vi "CAN_init.vi"(6 "error in":errorcluster, 8 "Maximum Output Voltage":dbl=5.0, 9 "Control Mode":T3=enum."Position") -> (0 "error out":errorcluster, 3 "CAN Jaguars Ref":T1)   [LabVIEW 2009, in "OWNCAN.lvlib"]
doc: "Initializes CAN interface for both Jaguars. Sets the default settings for controller parameters and enables corresponding control mode.\nThis VI must be called at the beginning of the program before using of any CAN functionality."
uses:
  OWNCAN.lvlib
  CAN/SubVIs/CAN Jaguar Control Mode.ctl
  CAN Jaguars Ref.ctl
  CAN/SubVIs/CAN Jaguar Ref.ctl
  CAN/SubVIs/CAN Jaguar Position Reference.ctl
  Serial.lvlib
  CAN.lvlib
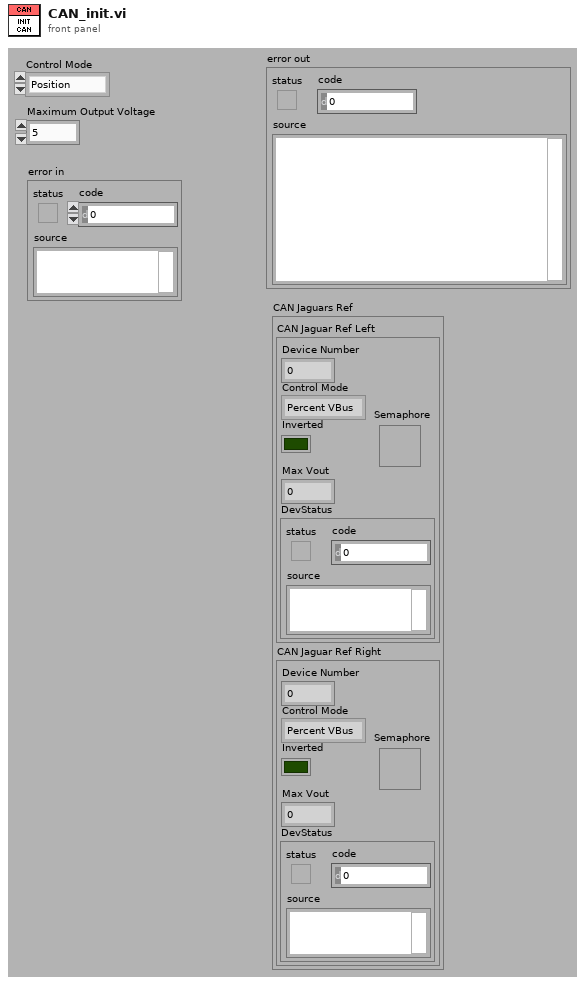
[diagram p1: front panel]
types:
  T1 = typedef "OWNCAN.lvlib/CAN Jaguars Ref.ctl" = cluster{"CAN Jaguar Ref Left":T2, "CAN Jaguar Ref Right":T2}
  T2 = typedef "CAN.lvlib/CAN Jaguar Ref.ctl" = cluster{"Device Number":u8, "Control Mode":T3, "Inverted":bool, "Semaphore":T4, "Max Vout":dbl, "DevStatus":errorcluster}
  T3 = typedef "CAN.lvlib/CAN Jaguar Control Mode.ctl" = enum16{"Percent VBus", "Speed", "Position", "Current"}
  T4 = typedef "Semaphore RefNum" = refnum<k1>
  T5 = typedef "CAN.lvlib/CAN Jaguar Position Reference.ctl" = enum16{"Encoder", "Potentiometer"}
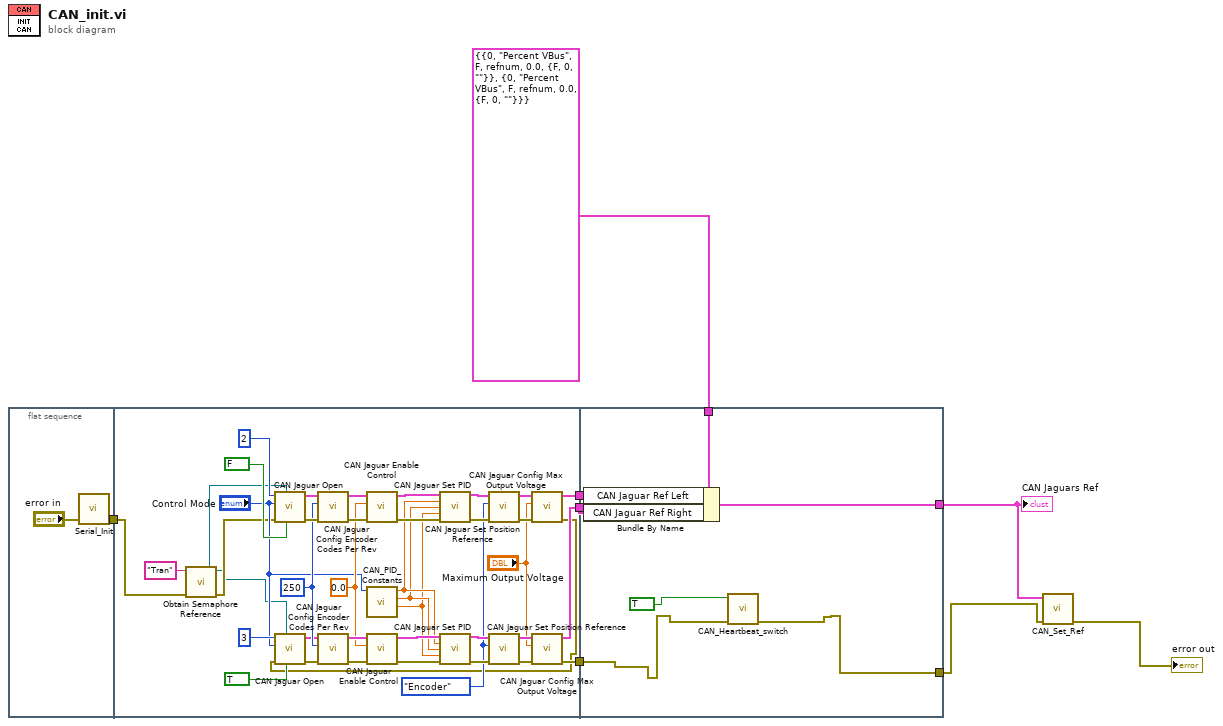
[diagram p0: block diagram]
diagram:
  n1 = flat-sequence {
    tunnel: [w9] -> w8
    tunnel: w8 -> [w15]
    tunnel: [w26] -> w7
    tunnel: [w25] -> w6
    tunnel: [w24] -> w5
    tunnel: w7 -> [w52]
    tunnel: w6 -> [w56]
    tunnel: w5 -> [w57]
    tunnel: [w55] -> w3
    tunnel: T1 {"CAN Jaguar Ref Left"={"Device Number"=0, "Control Mode"=enum."Percent VBus", "Inverted"=FALSE, "Semaphore"=refnum, "Max Vout"=0.0, "DevStatus"={"status"=FALSE, "code"=0, "source"=""}}, "CAN Jaguar Ref Right"={"Device Number"=0, "Control Mode"=enum."Percent VBus", "Inverted"=FALSE, "Semaphore"=refnum, "Max Vout"=0.0, "DevStatus"={"status"=FALSE, "code"=0, "source"=""}}} ("CAN Jaguars Ref") -> [w54]
    tunnel: [w51] -> w2
    frame #0 {
      n2 = call "Serial_Init.vi"("error in (no error)"="error in") -> ("error out"=w9:errorcluster)  [unwired: 3 in, 1 out]
    }
    frame #1 {
      w32 = 0.0 ("Encoder Initial Position")
      w33 = CAN_Jaguar_Position_Reference."Encoder" ("Position Reference")
      w46 = u16 250 ("Encoder Codes Per Rev")
      n3 = call <vilib>:"Obtain Semaphore Reference.vi"("error in (no error)"=w15, "name (unnamed)"="Tran") -> ("error out"=w14:errorcluster, "semaphore"=w11:T4)  [unwired: 3 in, 1 out]
      n4 = call "CAN Jaguar Open.vi"("Inverted"=FALSE, "Semaphore"=w11, "error in (no error)"=w14, "Control Mode"="Control Mode", "Device Number"=u8 2) -> ("error out"=w47:errorcluster, "CAN Jaguar Ref Out"=w12:T2)  [unwired: 5 in]
      n5 = call "CAN Jaguar Config Encoder Codes Per Rev.vi"("error in (no error)"=w47, "Encoder Codes Per Rev"=w46, "CAN Jaguar Ref"=w12) -> ("error out"=w43:errorcluster, "CAN Jaguar Ref Out"=w42:T2)  [unwired: 7 in]
      n6 = call "CAN Jaguar Enable Control.vi"("error in (no error)"=w43, "Encoder Initial Position"=w32, "CAN Jaguar Ref"=w42) -> ("error out"=w39:errorcluster, "CAN Jaguar Ref Out"=w41:T2)  [unwired: 7 in]
      n7 = call "CAN_PID_Constants.vi"("Control Mode"="Control Mode") -> ("D"=w18:dbl, "I"=w19:dbl, "P"=w20:dbl)  [unwired: 8 in]
      n8 = call "CAN Jaguar Set PID.vi"("CAN Jaguar Ref"=w41, "P"=w20, "I"=w19, "D"=w18, "error in (no error)"=w39) -> ("CAN Jaguar Ref Out"=w37:T2, "error out"=w36:errorcluster)  [unwired: 9 in]
      n9 = call "CAN Jaguar Set Position Reference.vi"("error in (no error)"=w36, "Position Reference"=w33, "CAN Jaguar Ref"=w37) -> ("error out"=w29:errorcluster, "CAN Jaguar Ref Out"=w30:T2)  [unwired: 7 in]
      n10 = call "CAN Jaguar Config Max Output Voltage.vi"("error in (no error)"=w29, "Maximum Output Voltage"="Maximum Output Voltage", "CAN Jaguar Ref"=w30) -> ("error out"=w17:errorcluster, "CAN Jaguar Ref Out"=w24:T2)  [unwired: 7 in]
      n11 = call "CAN Jaguar Open.vi"("Inverted"=TRUE, "Semaphore"=w11, "error in (no error)"=w17, "Control Mode"="Control Mode", "Device Number"=u8 3) -> ("error out"=w48:errorcluster, "CAN Jaguar Ref Out"=w13:T2)  [unwired: 5 in]
      n12 = call "CAN Jaguar Config Encoder Codes Per Rev.vi"("error in (no error)"=w48, "Encoder Codes Per Rev"=w46, "CAN Jaguar Ref"=w13) -> ("error out"=w45:errorcluster, "CAN Jaguar Ref Out"=w44:T2)  [unwired: 7 in]
      n13 = call "CAN Jaguar Enable Control.vi"("error in (no error)"=w45, "Encoder Initial Position"=w32, "CAN Jaguar Ref"=w44) -> ("error out"=w38:errorcluster, "CAN Jaguar Ref Out"=w40:T2)  [unwired: 7 in]
      n14 = call "CAN Jaguar Set PID.vi"("CAN Jaguar Ref"=w40, "P"=w20, "I"=w19, "D"=w18, "error in (no error)"=w38) -> ("CAN Jaguar Ref Out"=w35:T2, "error out"=w34:errorcluster)  [unwired: 9 in]
      n15 = call "CAN Jaguar Set Position Reference.vi"("error in (no error)"=w34, "Position Reference"=w33, "CAN Jaguar Ref"=w35) -> ("error out"=w28:errorcluster, "CAN Jaguar Ref Out"=w31:T2)  [unwired: 7 in]
      n16 = call "CAN Jaguar Config Max Output Voltage.vi"("error in (no error)"=w28, "Maximum Output Voltage"="Maximum Output Voltage", "CAN Jaguar Ref"=w31) -> ("error out"=w26:errorcluster, "CAN Jaguar Ref Out"=w25:T2)  [unwired: 7 in]
    }
    frame #2 {
      n17 = Bundle By Name(cluster=w54, "CAN Jaguar Ref Left"=w57, "CAN Jaguar Ref Right"=w56) -> (w55:T1)
      n18 = call "CAN_Heartbeat_switch.vi"("error in"=w52, "Enable? (T)"=TRUE ("CAN_Hearbeat_boolVar")) -> ("error out"=w51:errorcluster)  [unwired: 9 in]
    }
  }
  n19 = call "CAN_Set_Ref.vi"("error in (no error)"=w2, "CAN_Jaguars_ref"=w3) -> ("error out"=→"error out":errorcluster)  [unwired: 9 in]
  "CAN Jaguars Ref" <- w3
